vi "Model_Thickness.vi"() -> (5 "Plug in titles":string[](array[string]), 7 "Plug in values":string[](array[string]))   [LabVIEW 2020]
uses:
  Globals/Meas_global.vi
  Globals/Constants_global.vi
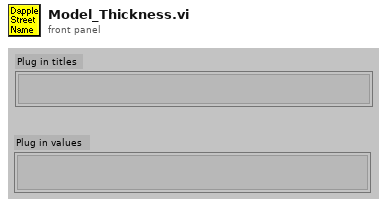
[diagram p1: front panel]
types:
  T1 = enum16{"To Traverse Coordinates", "To User Coordinates"}
  T2 = typedef "Post_Process.ctl" = enum16{"Take New Data", "Post Process Raw Data File"}
  T3 = typedef "Ch_description_ADAM.ctl" = cluster{"Ch Name":string, "Type":T4, "Function":T5, "Ch State":T6, "Calibration type":T7, "A":dbl, "B":dbl, "C":dbl, "D":dbl, "Comments":string, "Address":T8, "String":string, "Duty":u16}
  T4 = typedef "Module_type_ADAM.ctl" = string
  T5 = typedef "Function_ADAM.ctl" = enum16{"Analogue Input", "Digital Input", "Event counter", "Event rate", "Analogue Output", "Digital Output", "Relay Output"}
  T6 = typedef "Channel_State.ctl" = enum16{"On", "Off", "Always On", "Always Off"}
  T7 = typedef "Calib_type_ADAM.ctl" = string
  T8 = typedef "Address.ctl" = cluster{"Main":i32, "Ch.":i32, "Sub":i32, "Port Name":string}
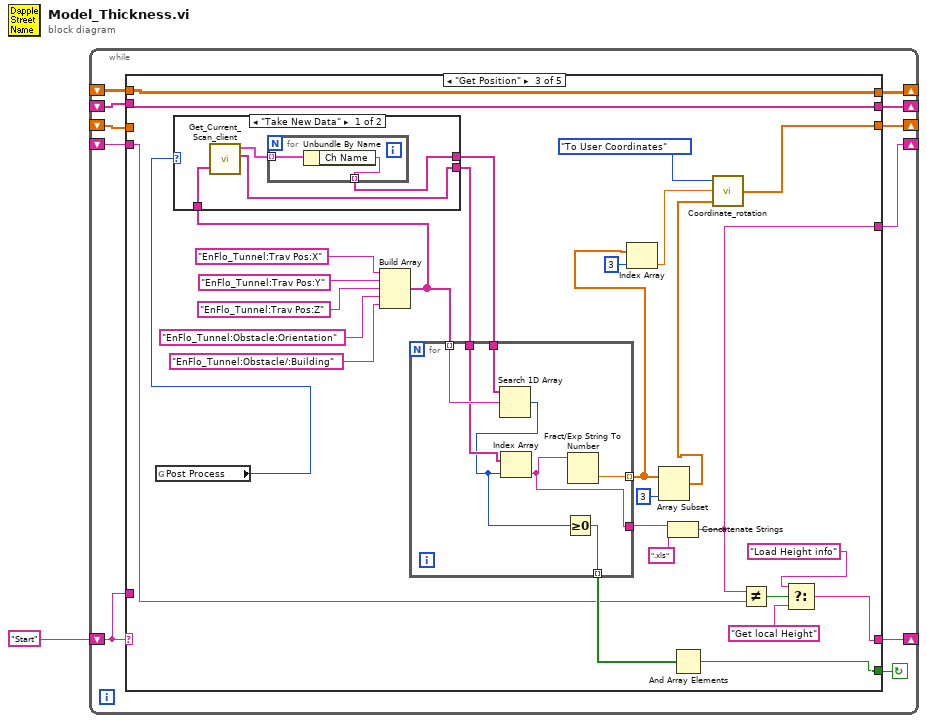
[diagram p0: block diagram]
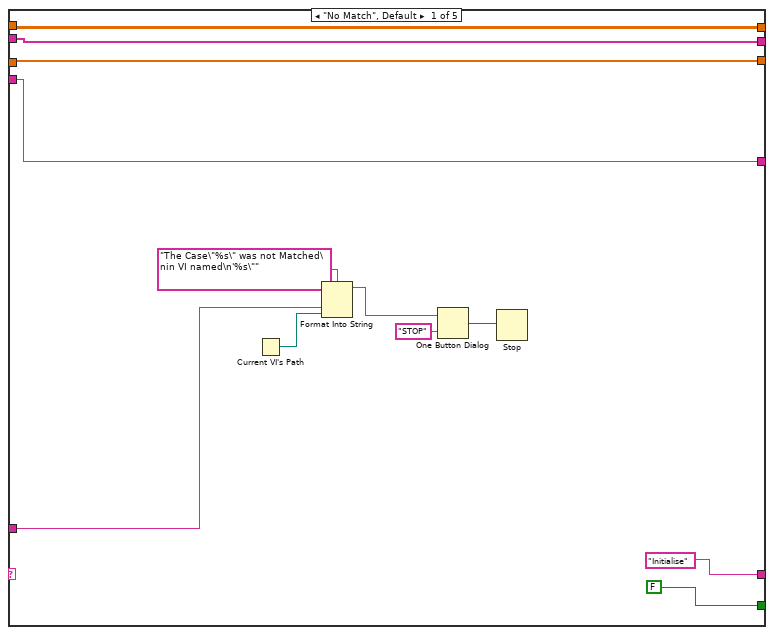
[diagram p2: hidden frame]
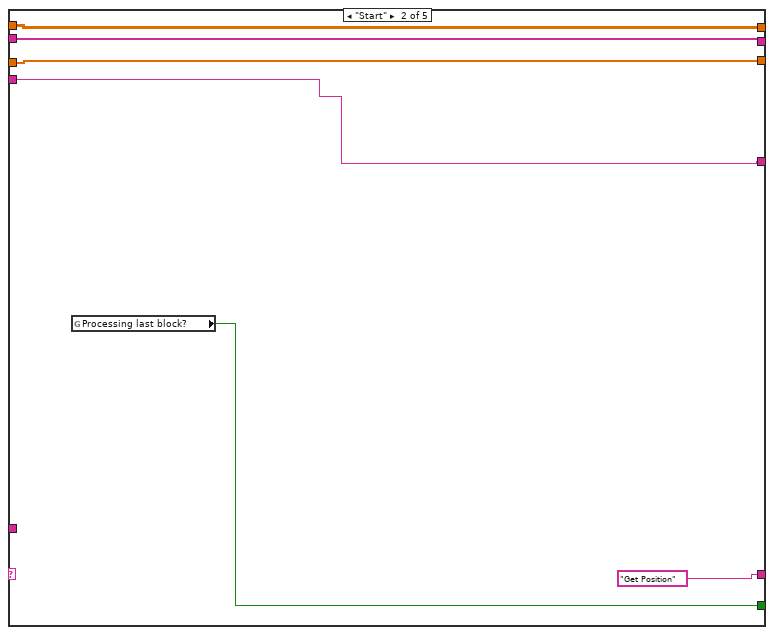
[diagram p3: hidden frame]
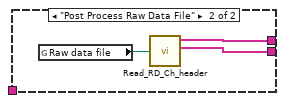
[diagram p4: hidden frame]
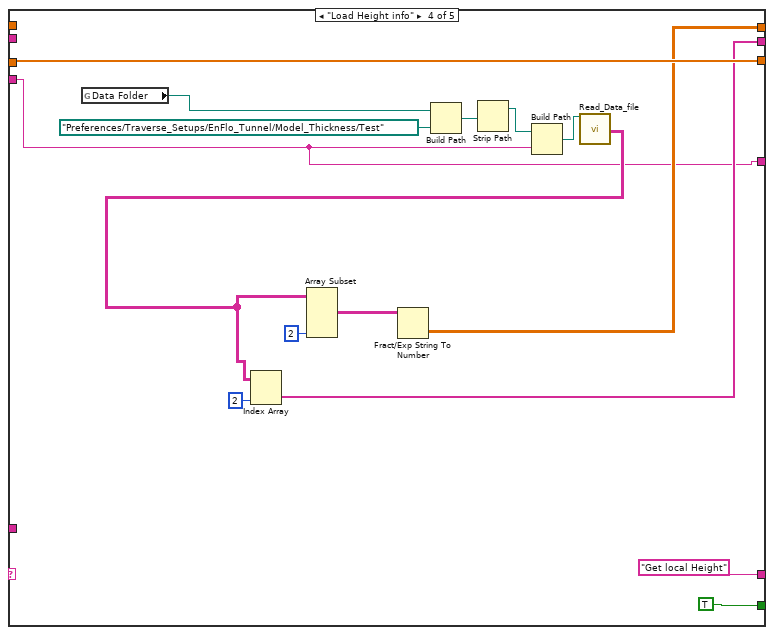
[diagram p5: hidden frame]
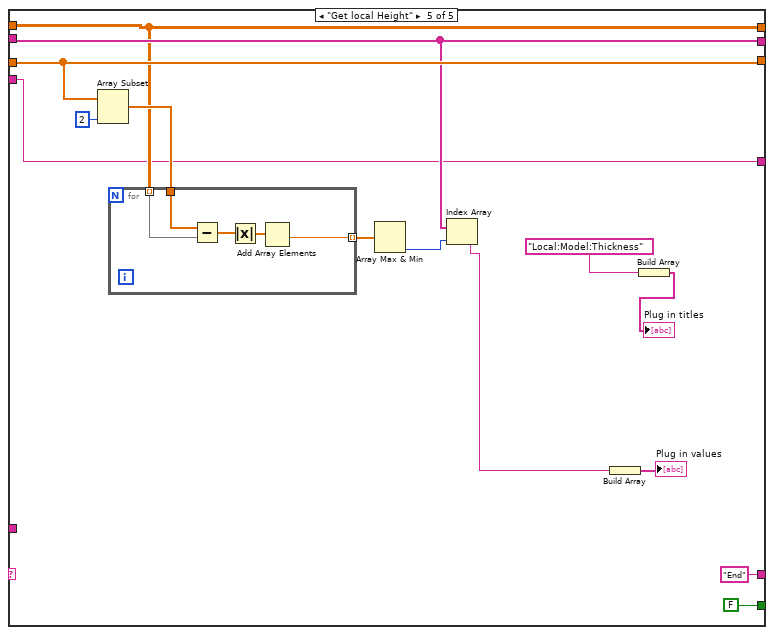
[diagram p6: hidden frame]
diagram:
  n1 = while {
    shift-left: "Start" -> [w10]
    shift-right: [w11] -> _
    shift-right: [w9] -> _
    shift-left: _ -> [w8]
    shift-right: [w7] -> _
    shift-left: _ -> [w6]
    shift-right: [w4] -> _
    shift-left: _ -> [w5]
    shift-right: [w3] -> _
    shift-left: _ -> [w2]
    stop <- w12 continue-if-true
    n2 = case shown="\"Get Position\"" w10 {
      tunnel: [FALSE w29 w48 TRUE FALSE ("Processing last block?")] -> w12
      tunnel: ["Initialise" "Get Position" w36 "Get local Height" "End"] -> w11
      tunnel: w10 -> [w19 _ _ _ _]
      tunnel: [w16 w28 w57 w82 w93] -> w9
      tunnel: w8 -> [w16 w28 w57 _ w93]
      tunnel: [w15 w30 w58 w85 w98] -> w7
      tunnel: w6 -> [w15 w30 _ w85 w98]
      tunnel: [w14 w25 w34 w80 w92] -> w3
      tunnel: w5 -> [w13 w27 w39 w75 w90]
      tunnel: [w13 w27 w32 w75 w90] -> w4
      tunnel: w2 -> [w14 w25 w34 _ w92]
      frame "No Match", Default {
        n3 = Current VI's Path() -> (path=w18:path)
        n4 = Format Into String(format string="The Case\"%s\" was not Matched\nin VI named\n'%s\"" ("Format String"), w19, w18) -> (resulting string=w22:string)  [unwired: 2 in, 1 out]
        n5 = One Button Dialog(message=w22, button name ("OK")="STOP") -> (true=w20:bool)
        n6 = Stop(stop? (T)=w20) -> ()
      }
      frame "Start" {
        n7 = global read "Meas_global.vi" "Processing last block?"() -> (w29:bool)
      }
      frame "Get Position" {
        n8 = global read "Meas_global.vi" "Post Process"() -> (w42:T2)
        n9 = Build Array("EnFlo_Tunnel:Trav Pos:X", "EnFlo_Tunnel:Trav Pos:Y", "EnFlo_Tunnel:Trav Pos:Z", "EnFlo_Tunnel:Obstacle:Orientation", "EnFlo_Tunnel:Obstacle/:Building") -> (w41:string[])
        n10 = case shown="\"Take New Data\"" w42 {
          tunnel: [w61 w66] -> w51
          tunnel: [w60 w65] -> w50
          tunnel: w41 -> [w59 _]
          frame "Take New Data" {
            n11 = call "Get_Current_Scan_client.vi"("multipleChannels"=w59) -> ("Ch Description Array"=w62:T3[], "String values"=w60:string[])  [unwired: 2 in, 1 out]
            n12 = for {
              tunnel: w62 -> [w64] mode=indexing
              tunnel: [w63] -> w61 mode=indexing
              n13 = Unbundle By Name(w64) -> ("Ch Name"=w63:string)
            }
          }
          frame "Post Process Raw Data File" {
            n14 = global read "Meas_global.vi" "Raw data file"() -> (w67:path)
            n15 = call "Read_RD_Ch_header.vi"("Raw data file"=w67) -> ("Ch Name Out"=w66:string[], "Ch Values"=w65:string[])  [unwired: 2 out]
          }
        }
        n16 = for {
          tunnel: [w74] -> w43 mode=indexing
          tunnel: w41 -> [w73] mode=indexing
          tunnel: w51 -> [w72]
          tunnel: w50 -> [w71]
          tunnel: [w69] -> w49 mode=indexing
          tunnel: [w68] -> w33
          n17 = Search 1D Array(1D array=w72, element=w73) -> (index of element=w70:i32)  [unwired: 1 out]
          n18 = Index Array(array=w71, index=w70) -> (element=w68:string)
          n19 = Greater Or Equal To 0?(x=w70) -> (x >= 0?=w69:bool)
          n20 = Fract/Exp String To Number(string=w68) -> (number=w74:dbl)  [unwired: 4 out]
        }
        n21 = Index Array(array=w43, index=3) -> (element=w46:dbl)
        n22 = Array Subset(array=w43, length=3) -> (w44:dbl[])  [unwired: 1 in]
        n23 = Concatenate Strings(w33, ".xls" ("string")) -> (w32:string)
        n24 = And Array Elements(Boolean array=w49) -> (logical AND=w48:bool)
        n25 = call "Coordinate_rotation.vi"("Input Position"=w44, "Coordinate rotation (deg)"=w46, "Mode"=T1."To User Coordinates") -> ("Output Position"=w58:dbl[])
        n26 = Not Equal?(x=w32, y=w39) -> (x != y?=w37:bool)
        n27 = Select(t="Load Height info", s=w37, f="Get local Height") -> (s? t:f=w36:string)
      }
      frame "Load Height info" {
        n28 = global read "Constants_global.vi" "Data Folder"() -> (w87:path)
        n29 = Build Path(base path=w87, name or relative path=path "Preferences/Traverse_Setups/EnFlo_Tunnel/Model_Thickness/Test") -> (appended path=w78:path)
        n30 = Strip Path(path=w78) -> (stripped path=w77:path)  [unwired: 1 out]
        n31 = Build Path(base path=w77, name or relative path=w75) -> (appended path=w76:path)
        n32 = call "Read_Data_file.vi"("Results file"=w76) -> ("Channel Values Out"=w79:string[][])  [unwired: 6 in, 12 out]
        n33 = Index Array(array=w79, index (col)=2 ("disabled index (col)")) -> (element=w82:string[])  [unwired: 1 in]
        n34 = Array Subset(array=w79, length (col)=2 ("length")) -> (w81:string[][])  [unwired: 3 in]
        n35 = Fract/Exp String To Number(string=w81) -> (number=w80:dbl[][])  [unwired: 4 out]
      }
      frame "Get local Height" {
        n36 = Array Subset(array=w98, length=2) -> (w96:dbl[])  [unwired: 1 in]
        n37 = for {
          tunnel: w96 -> [w108]
          tunnel: w92 -> [w107] mode=indexing
          tunnel: [w104] -> w95 mode=indexing
          n38 = Subtract(x=w108, y=w107) -> (x-y=w106:dbl[])
          n39 = Absolute Value(x=w106) -> (abs(x)=w105:dbl[])
          n40 = Add Array Elements(numeric array=w105) -> (sum=w104:dbl)
        }
        n41 = Array Max & Min(array=w95) -> (min index (indices)=w94:i32)  [unwired: 3 out]
        n42 = Index Array(array=w93, index=w94) -> (element=w91:string)
        n43 = Build Array(w91) -> (→"Plug in values":string[])
        n44 = Build Array("Local:Model:Thickness") -> (→"Plug in titles":string[])
      }
    }
  }
